vi "tb_complex multiplier.vi"() -> ()   [LabVIEW 2011]
panel:
  out "FLP Complex Multiply":cdb
  out "Imag Error":dbl=2.6275520212948322e-06
  out "Real Error":dbl=7.476774044334888e-07
  out "Imag":dbl[](array[numeric])=[0.0652008056640625, 0.0652008056640625, 0.0652008056640625, 0.0652008056640625, 0.0652008056640625, 0.0652008056640625] format="%#.5f"
  out "Real":dbl[](array[numeric])=[-0.00099945068359375, -0.00099945068359375, -0.00099945068359375, -0.00099945068359375, -0.00099945068359375, -0.00099945068359375] format="%#.5f"
  in  "Imag{Twiddle}":fxp<+/-,18,1>=0.23999786376953125 format="%.6f"
  in  "Real{Twiddle}":fxp<+/-,18,1>=0.09999847412109375 format="%.6f"
  in  "Imag{Input}":fxp<+/-,18,1>=0.09999847412109375
  in  "Real{Input}":fxp<+/-,18,1>=0.2299957275390625
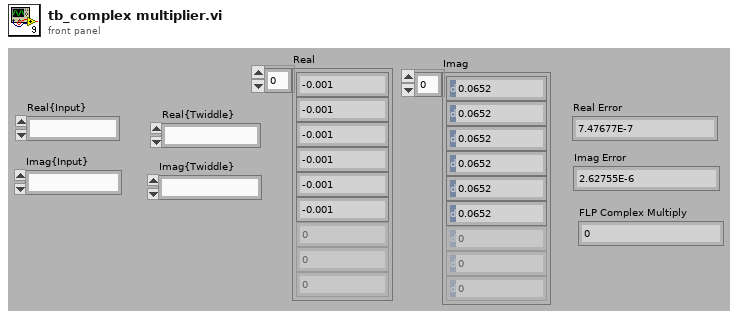
[diagram p1: front panel]
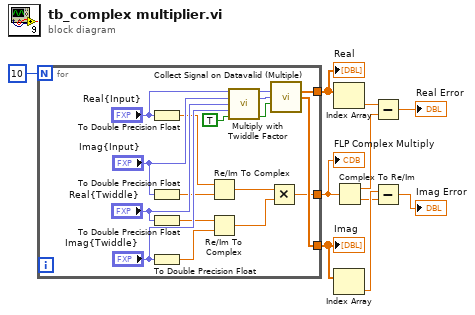
[diagram p0: block diagram]
diagram:
  n1 = for {
    N: 10 -> [_]
    tunnel: [w23] -> w9
    tunnel: [w22] -> w8
    tunnel: [w11] -> w7
    n2 = To Double Precision Float(number="Real{Input}") -> (double precision float=w17:dbl)
    n3 = To Double Precision Float(number="Imag{Input}") -> (double precision float=w16:dbl)
    n4 = To Double Precision Float(number="Real{Twiddle}") -> (double precision float=w15:dbl)
    n5 = To Double Precision Float(number="Imag{Twiddle}") -> (double precision float=w14:dbl)
    n6 = Re/Im To Complex(1:w16, 2:w17) -> (0:w13:cdb)
    n7 = Re/Im To Complex(1:w14, 2:w15) -> (0:w12:cdb)
    n8 = call "Multiply with Twiddle Factor.vi"("Real{Input}"="Real{Input}", "Imag{Input}"="Imag{Input}", "Real{Twiddle}"="Real{Twiddle}", "Imag{Twiddle}"="Imag{Twiddle}", "Input Valid"=TRUE) -> ("Real{Output}"=w26:fxp<+/-,19,2>, "Imag{Output}"=w25:fxp<+/-,19,2>, "Output Valid"=w24:bool)  [unwired: 8 in]
    n9 = Multiply(x=w13, y=w12) -> (x*y=w11:cdb)
    n10 = call <userlib>:"Collect Signal on Datavalid (Multiple).vi"("Input 1"=w26, "Input 2"=w25, "Data Valid"=w24) -> ("Output 1"=w23:dbl[], "Output 2"=w22:dbl[])  [unwired: 11 in]
  }
  "Real" <- w9
  "Imag" <- w8
  "FLP Complex Multiply" <- w7
  n11 = Index Array(array=w9) -> (element=w5:dbl)  [unwired: 1 in]
  n12 = Index Array(array=w8) -> (element=w3:dbl)  [unwired: 1 in]
  n13 = Complex To Re/Im(x + iy=w7) -> (x=w6:dbl, y=w2:dbl)
  n14 = Subtract(x=w5, y=w6) -> (x-y=→"Real Error":dbl)
  n15 = Subtract(x=w3, y=w2) -> (x-y=→"Imag Error":dbl)
